vi "MatrixSwitch.vi"(8 "error in (no error)":errorcluster, 10 "Action":T1(ring), 11 "Pickering in":refnum<class "Pickering.lvclass">) -> (0 "error out":errorcluster, 2 "Continue?":bool, 3 "Pickering out":refnum<class "Pickering.lvclass">)   [LabVIEW 2019, in "Pickering.lvclass"]
uses:
  Pickering.lvclass
  InstrumentSetup.vi
  InstrControl.lvclass
panel:
  out "Display Matrix":bool[][](array[boolean])
  # "Pickering Matrix Settings"
  # "X1"
  # "X2"
  # "X3"
  # "X4"
  # "X5"
  # "X6"
  # "X7"
  # "X8"
  # "X9"
  # "X10"
  # "X11"
  # "X12"
  # "Y1"
  # "Y2"
  # "Y3"
  # "Y4"
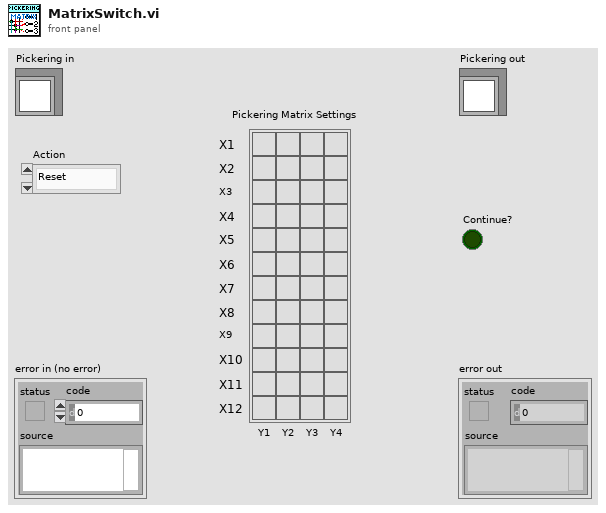
[diagram p1: front panel]
types:
  T1 = enum16{"Reset", "Ground", "Striptest Bias", "Striptest SMU", "Striptest LCR", "IV", "CV", "Interstrip Cap", "Interstrip Res", "PTP", "Implant Resistance", "Metal Resistance", "Coupling Capacitance"}
  T2 = cluster{"Matrix address":string, "Mux1 address":string, "Mux2 address":string, "Pickering":refnum<class "Pickering.lvclass">, "Matrix X Channels":cluster{"Bias Supply / SMU LO":i32, "Bias Supply / SMU HI":i32, "CV Box LO":i32, "CV Box HI":i32, "CV Box LO IN":i32, "CV Box HI IN":i32, "Volt meter LO":i32, "Volt meter HI":i32, "Mux1 C1":i32, "Mux1 C2":i32, "Mux2 C1":i32, "Mux2 C2":i32}}
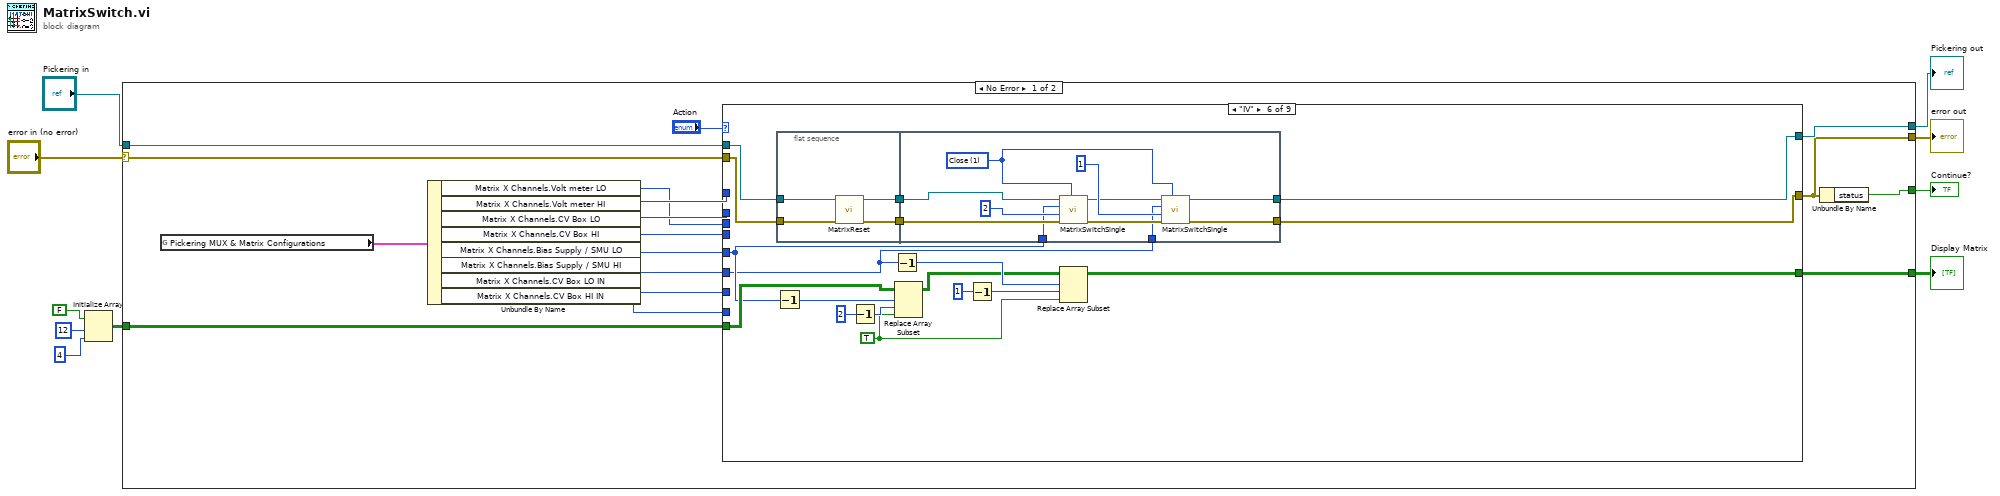
[diagram p0: block diagram]
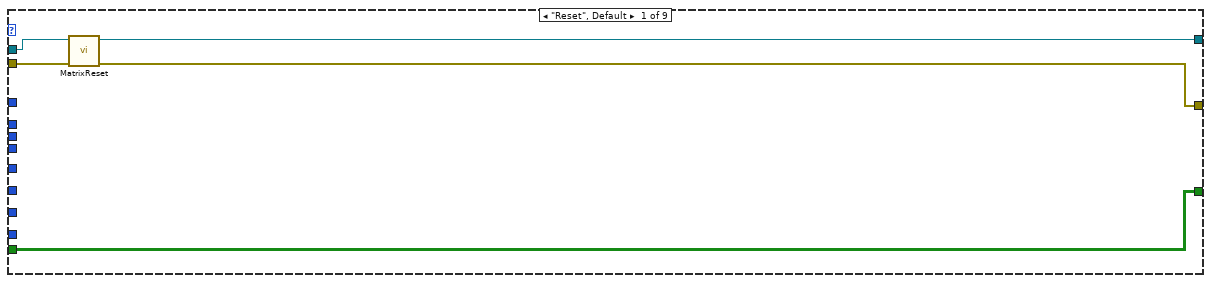
[diagram p2: hidden frame]
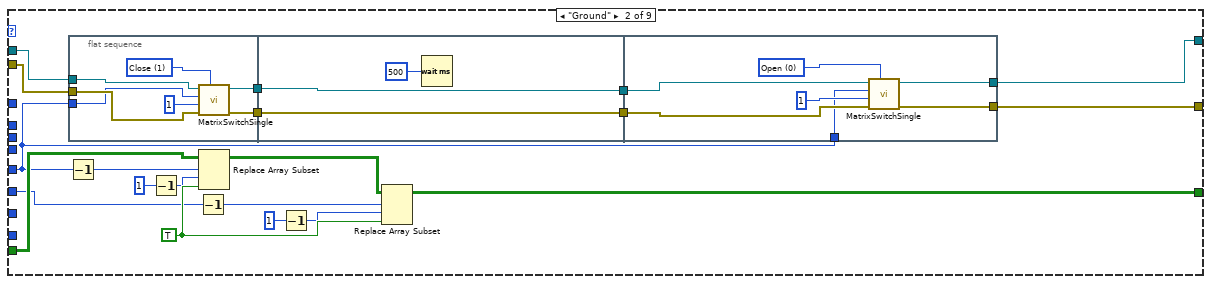
[diagram p3: hidden frame]
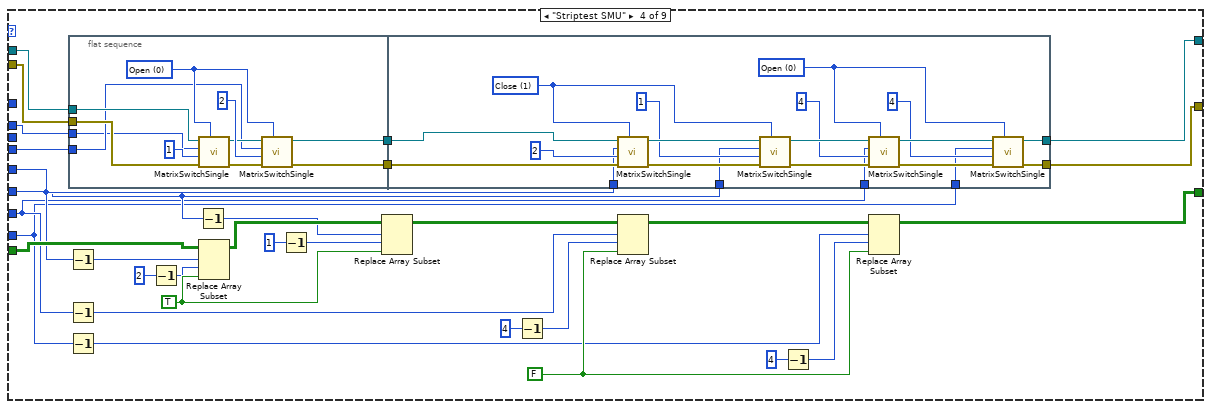
[diagram p5: hidden frame]
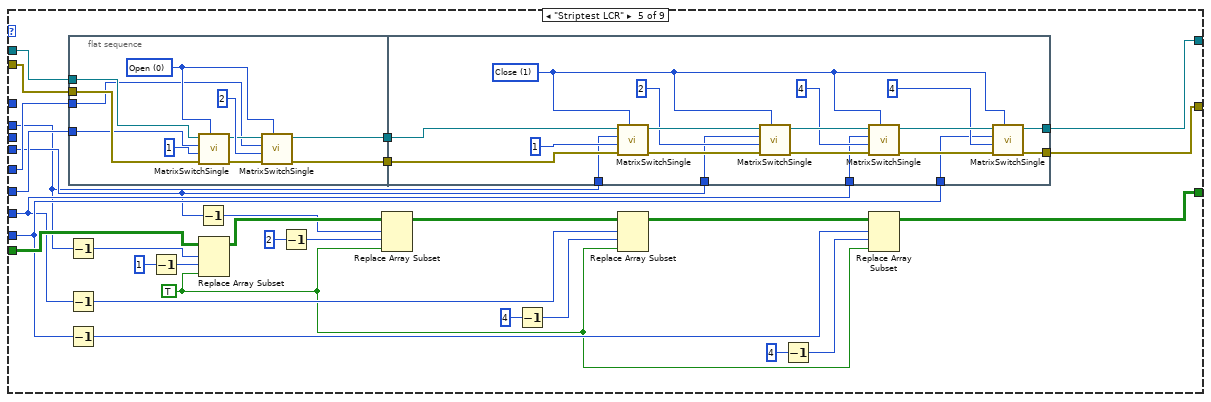
[diagram p6: hidden frame]
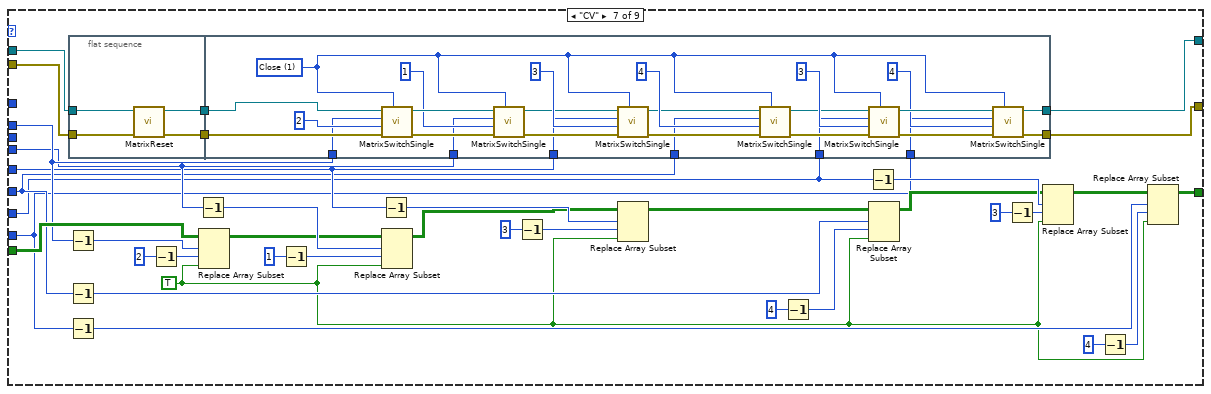
[diagram p7: hidden frame]
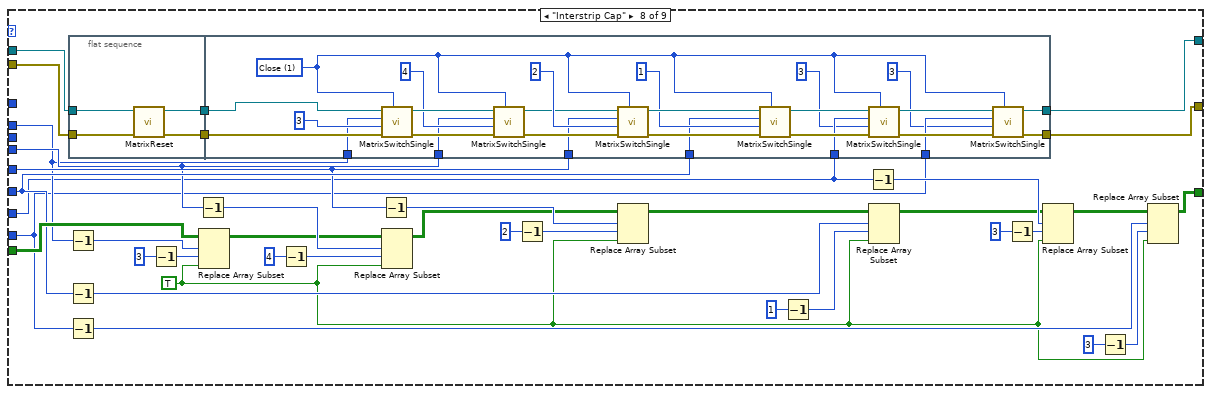
[diagram p8: hidden frame]
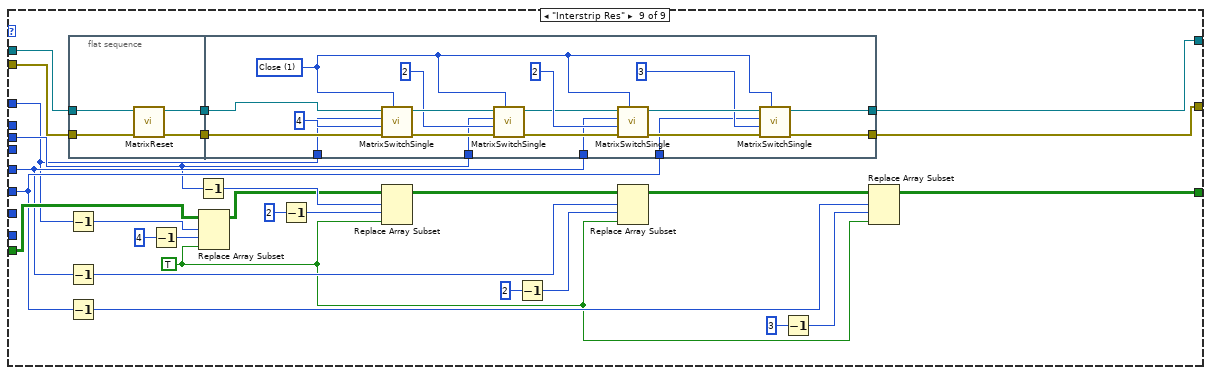
[diagram p9: hidden frame]
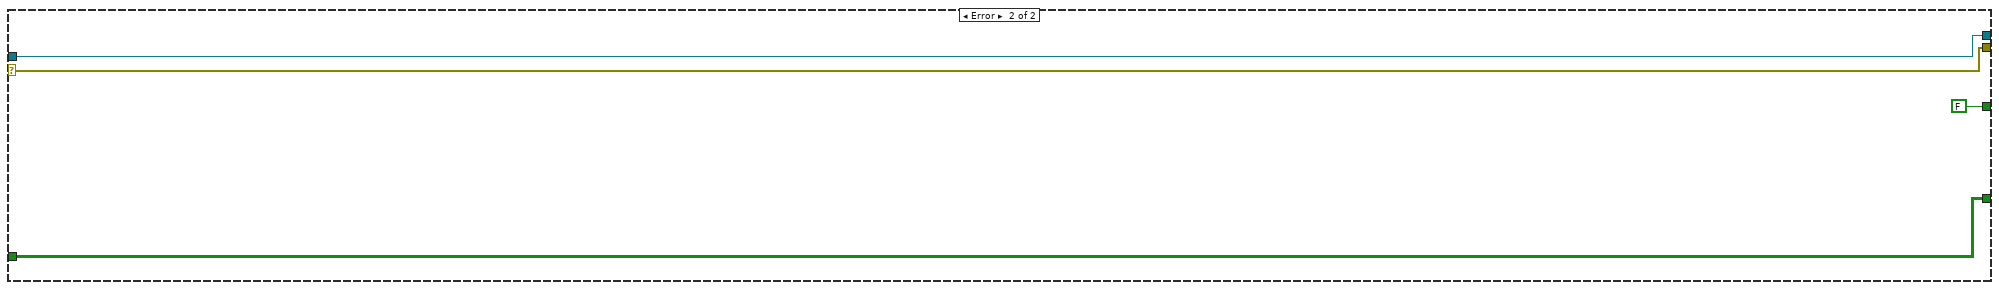
[diagram p10: hidden frame]
diagram:
  n1 = Initialize Array(FALSE, 12, 4) -> (w5:bool[][])
  n2 = case shown="No Error" "error in (no error)" {
    selector: "error in (no error)" -> [w21 w420]
    tunnel: [w24 w420] -> w2
    tunnel: [w25 w419] -> w1
    tunnel: "Pickering in" -> [w22 w419]
    tunnel: [w23 FALSE] -> w4
    tunnel: w5 -> [w27 w417]
    tunnel: [w26 w417] -> w3
    frame No Error {
      n3 = global read "InstrumentSetup.vi" "Pickering MUX & Matrix Configurations"() -> (w20:T2)
      n4 = Unbundle By Name(w20) -> ("Matrix X Channels.Volt meter LO"=w14:i32, "Matrix X Channels.Volt meter HI"=w15:i32, "Matrix X Channels.CV Box LO"=w19:i32, "Matrix X Channels.CV Box HI"=w18:i32, "Matrix X Channels.Bias Supply / SMU LO"=w12:i32, "Matrix X Channels.Bias Supply / SMU HI"=w13:i32, "Matrix X Channels.CV Box LO IN"=w17:i32, "Matrix X Channels.CV Box HI IN"=w16:i32)
      n5 = case shown="\"IV\"" "Action" {
        tunnel: w27 -> [w32 w37 w72 w90 w153 w203 w240 w320 w378]
        tunnel: [w32 w35 w72 w89 w152 w204 w241 w297 w379] -> w26
        tunnel: w21 -> [w29 w52 w71 w79 w142 w211 w239 w319 w377]
        tunnel: w22 -> [w31 w49 w70 w81 w141 w212 w238 w318 w376]
        tunnel: [w30 w46 w70 w84 w147 w200 w234 w314 w372] -> w25
        tunnel: [w28 w45 w71 w83 w146 w199 w235 w315 w373] -> w24
        tunnel: w12 -> [_ w34 _ w76 w139 w196 w231 w311 w368]
        tunnel: w13 -> [_ w33 _ w75 w140 w195 w230 w312 w369]
        tunnel: w19 -> [_ _ _ w77 w135 _ w233 w309 _]
        tunnel: w18 -> [_ _ _ w78 w136 _ w232 w310 _]
        tunnel: w17 -> [_ _ _ w74 w137 _ w229 w301 _]
        tunnel: w16 -> [_ _ _ w73 w138 _ w228 w300 _]
        tunnel: w14 -> [_ _ _ _ _ _ _ _ w367]
        tunnel: w15 -> [_ _ _ _ _ _ _ _ w366]
        frame "Reset", Default {
          n6 = call-dynamic "MatrixReset.vi"("error in (no error)"=w29, "Pickering in"=w31) -> ("error out"=w28:errorcluster, "Pickering out"=w30:refnum<class "Pickering.lvclass">)  [unwired: 8 in]
        }
        frame "Ground" {
          w43 = TRUE
          n7 = Decrement(x=w34) -> (x-1=w38:i32)
          n8 = flat-sequence {
            tunnel: w52 -> [w57]
            tunnel: [w56] -> w51
            tunnel: w49 -> [w55]
            tunnel: [w54] -> w47
            tunnel: w34 -> [w53]
            tunnel: w51 -> [w61]
            tunnel: [w61] -> w50
            tunnel: [w60] -> w48
            tunnel: w47 -> [w60]
            tunnel: w50 -> [w68]
            tunnel: w48 -> [w66]
            tunnel: [w65] -> w46
            tunnel: [w64] -> w45
            tunnel: w34 -> [w63]
            frame #0 {
              w59 = u16 1 items=["Open", "Close"] ("Switch action")
              n9 = call-dynamic "MatrixSwitchSingle.vi"("Switch action"=w59, "error in (no error)"=w57, "Matrix Y"=1, "Matrix X"=w53, "Pickering in"=w55) -> ("error out"=w56:errorcluster, "Pickering out"=w54:refnum<class "Pickering.lvclass">)  [unwired: 4 in, 1 out]
            }
            frame #1 {
              n10 = Wait (ms)(milliseconds to wait=u32 500) -> ()  [unwired: 1 out]
            }
            frame #2 {
              w69 = u16 0 items=["Open", "Close"] ("Switch action")
              n11 = call-dynamic "MatrixSwitchSingle.vi"("Switch action"=w69, "error in (no error)"=w68, "Matrix Y"=1, "Matrix X"=w63, "Pickering in"=w66) -> ("error out"=w64:errorcluster, "Pickering out"=w65:refnum<class "Pickering.lvclass">)  [unwired: 4 in, 1 out]
            }
          }
          n12 = Decrement(x=1 ("Matrix Y")) -> (x-1=w39:i32)
          n13 = Decrement(x=w33) -> (x-1=w40:i32)
          n14 = Replace Array Subset(array=w37, new element=w43, index (row)=w38, index (col)=w39) -> (w44:bool[][])
          n15 = Decrement(x=1 ("Matrix Y")) -> (x-1=w41:i32)
          n16 = Replace Array Subset(array=w44, new element=w43, index (row)=w40, index (col)=w41) -> (w35:bool[][])
        }
        frame "Striptest Bias" {
          # "Does nothing as the bias is connected directly for the Pickering GPIB switching system."
        }
        frame "Striptest SMU" {
          w103 = FALSE
          w102 = TRUE
          n17 = Decrement(x=w76) -> (x-1=w92:i32)
          n18 = Decrement(x=w74) -> (x-1=w97:i32)
          n19 = Decrement(x=w73) -> (x-1=w98:i32)
          n20 = flat-sequence {
            tunnel: [w110] -> w82
            tunnel: w81 -> [w108]
            tunnel: [w107] -> w80
            tunnel: w79 -> [w106]
            tunnel: w78 -> [w105]
            tunnel: w77 -> [w104]
            tunnel: [w123] -> w84
            tunnel: [w122] -> w83
            tunnel: w82 -> [w120]
            tunnel: w80 -> [w119]
            tunnel: w74 -> [w118]
            tunnel: w73 -> [w117]
            tunnel: w75 -> [w116]
            tunnel: w76 -> [w115]
            frame #0 {
              w109 = u16 0 items=["Open", "Close"] ("Switch action")
              n21 = call-dynamic "MatrixSwitchSingle.vi"("Switch action"=w109, "error in (no error)"=w106, "Matrix Y"=1, "Matrix X"=w104, "Pickering in"=w108) -> ("error out"=w113:errorcluster, "Pickering out"=w112:refnum<class "Pickering.lvclass">)  [unwired: 4 in, 1 out]
              n22 = call-dynamic "MatrixSwitchSingle.vi"("Switch action"=w109, "error in (no error)"=w113, "Matrix Y"=2, "Matrix X"=w105, "Pickering in"=w112) -> ("error out"=w110:errorcluster, "Pickering out"=w107:refnum<class "Pickering.lvclass">)  [unwired: 4 in, 1 out]
            }
            frame #1 {
              w121 = u16 0 items=["Open", "Close"] ("Switch action")
              w132 = u16 1 items=["Open", "Close"] ("Switch action")
              n23 = call-dynamic "MatrixSwitchSingle.vi"("Switch action"=w132, "error in (no error)"=w120, "Matrix Y"=2, "Matrix X"=w115, "Pickering in"=w119) -> ("error out"=w130:errorcluster, "Pickering out"=w133:refnum<class "Pickering.lvclass">)  [unwired: 4 in, 1 out]
              n24 = call-dynamic "MatrixSwitchSingle.vi"("Switch action"=w132, "error in (no error)"=w130, "Matrix Y"=1, "Matrix X"=w116, "Pickering in"=w133) -> ("error out"=w128:errorcluster, "Pickering out"=w129:refnum<class "Pickering.lvclass">)  [unwired: 4 in, 1 out]
              n25 = call-dynamic "MatrixSwitchSingle.vi"("Switch action"=w121, "error in (no error)"=w128, "Matrix Y"=4, "Matrix X"=w118, "Pickering in"=w129) -> ("error out"=w125:errorcluster, "Pickering out"=w126:refnum<class "Pickering.lvclass">)  [unwired: 4 in, 1 out]
              n26 = call-dynamic "MatrixSwitchSingle.vi"("Switch action"=w121, "error in (no error)"=w125, "Matrix Y"=4, "Matrix X"=w117, "Pickering in"=w126) -> ("error out"=w122:errorcluster, "Pickering out"=w123:refnum<class "Pickering.lvclass">)  [unwired: 4 in, 1 out]
            }
          }
          n27 = Decrement(x=2 ("Matrix Y")) -> (x-1=w91:i32)
          n28 = Decrement(x=w75) -> (x-1=w93:i32)
          n29 = Replace Array Subset(array=w90, new element=w102, index (row)=w92, index (col)=w91) -> (w95:bool[][])
          n30 = Decrement(x=1 ("Matrix Y")) -> (x-1=w94:i32)
          n31 = Replace Array Subset(array=w95, new element=w102, index (row)=w93, index (col)=w94) -> (w101:bool[][])
          n32 = Decrement(x=4 ("Matrix Y")) -> (x-1=w96:i32)
          n33 = Replace Array Subset(array=w101, new element=w103, index (row)=w97, index (col)=w96) -> (w100:bool[][])
          n34 = Decrement(x=4 ("Matrix Y")) -> (x-1=w99:i32)
          n35 = Replace Array Subset(array=w100, new element=w103, index (row)=w98, index (col)=w99) -> (w89:bool[][])
        }
        frame "Striptest LCR" {
          w145 = TRUE
          n36 = Decrement(x=w135) -> (x-1=w155:i32)
          n37 = Decrement(x=w137) -> (x-1=w160:i32)
          n38 = Decrement(x=w138) -> (x-1=w161:i32)
          n39 = flat-sequence {
            tunnel: [w171] -> w144
            tunnel: [w170] -> w143
            tunnel: w142 -> [w169]
            tunnel: w141 -> [w168]
            tunnel: w139 -> [w166]
            tunnel: w140 -> [w165]
            tunnel: [w184] -> w147
            tunnel: [w183] -> w146
            tunnel: w144 -> [w181]
            tunnel: w143 -> [w180]
            tunnel: w135 -> [w179]
            tunnel: w136 -> [w178]
            tunnel: w137 -> [w177]
            tunnel: w138 -> [w176]
            frame #0 {
              w167 = u16 0 items=["Open", "Close"] ("Switch action")
              n40 = call-dynamic "MatrixSwitchSingle.vi"("Switch action"=w167, "error in (no error)"=w169, "Matrix Y"=1, "Matrix X"=w165, "Pickering in"=w168) -> ("error out"=w174:errorcluster, "Pickering out"=w173:refnum<class "Pickering.lvclass">)  [unwired: 4 in, 1 out]
              n41 = call-dynamic "MatrixSwitchSingle.vi"("Switch action"=w167, "error in (no error)"=w174, "Matrix Y"=2, "Matrix X"=w166, "Pickering in"=w173) -> ("error out"=w170:errorcluster, "Pickering out"=w171:refnum<class "Pickering.lvclass">)  [unwired: 4 in, 1 out]
            }
            frame #1 {
              w182 = u16 1 items=["Open", "Close"] ("Switch action")
              n42 = call-dynamic "MatrixSwitchSingle.vi"("Switch action"=w182, "error in (no error)"=w180, "Matrix Y"=1, "Matrix X"=w179, "Pickering in"=w181) -> ("error out"=w191:errorcluster, "Pickering out"=w193:refnum<class "Pickering.lvclass">)  [unwired: 4 in, 1 out]
              n43 = call-dynamic "MatrixSwitchSingle.vi"("Switch action"=w182, "error in (no error)"=w191, "Matrix Y"=2, "Matrix X"=w178, "Pickering in"=w193) -> ("error out"=w189:errorcluster, "Pickering out"=w190:refnum<class "Pickering.lvclass">)  [unwired: 4 in, 1 out]
              n44 = call-dynamic "MatrixSwitchSingle.vi"("Switch action"=w182, "error in (no error)"=w189, "Matrix Y"=4, "Matrix X"=w177, "Pickering in"=w190) -> ("error out"=w186:errorcluster, "Pickering out"=w187:refnum<class "Pickering.lvclass">)  [unwired: 4 in, 1 out]
              n45 = call-dynamic "MatrixSwitchSingle.vi"("Switch action"=w182, "error in (no error)"=w186, "Matrix Y"=4, "Matrix X"=w176, "Pickering in"=w187) -> ("error out"=w183:errorcluster, "Pickering out"=w184:refnum<class "Pickering.lvclass">)  [unwired: 4 in, 1 out]
            }
          }
          n46 = Decrement(x=1 ("Matrix Y")) -> (x-1=w154:i32)
          n47 = Decrement(x=w136) -> (x-1=w156:i32)
          n48 = Replace Array Subset(array=w153, new element=w145, index (row)=w155, index (col)=w154) -> (w158:bool[][])
          n49 = Decrement(x=2 ("Matrix Y")) -> (x-1=w157:i32)
          n50 = Replace Array Subset(array=w158, new element=w145, index (row)=w156, index (col)=w157) -> (w164:bool[][])
          n51 = Decrement(x=4 ("Matrix Y")) -> (x-1=w159:i32)
          n52 = Replace Array Subset(array=w164, new element=w145, index (row)=w160, index (col)=w159) -> (w163:bool[][])
          n53 = Decrement(x=4 ("Matrix Y")) -> (x-1=w162:i32)
          n54 = Replace Array Subset(array=w163, new element=w145, index (row)=w161, index (col)=w162) -> (w152:bool[][])
        }
        frame "IV" {
          w206 = TRUE
          n55 = Decrement(x=w196) -> (x-1=w208:i32)
          n56 = flat-sequence {
            tunnel: w212 -> [w216]
            tunnel: w211 -> [w215]
            tunnel: [w214] -> w202
            tunnel: [w213] -> w201
            tunnel: w202 -> [w222]
            tunnel: w201 -> [w221]
            tunnel: [w220] -> w200
            tunnel: [w219] -> w199
            tunnel: w195 -> [w218]
            tunnel: w196 -> [w217]
            frame #0 {
              n57 = call-dynamic "MatrixReset.vi"("error in (no error)"=w215, "Pickering in"=w216) -> ("error out"=w213:errorcluster, "Pickering out"=w214:refnum<class "Pickering.lvclass">)  [unwired: 8 in]
            }
            frame #1 {
              w227 = u16 1 items=["Open", "Close"] ("Switch action")
              n58 = call-dynamic "MatrixSwitchSingle.vi"("Switch action"=w227, "error in (no error)"=w221, "Matrix Y"=2, "Matrix X"=w217, "Pickering in"=w222) -> ("error out"=w225:errorcluster, "Pickering out"=w224:refnum<class "Pickering.lvclass">)  [unwired: 4 in, 1 out]
              n59 = call-dynamic "MatrixSwitchSingle.vi"("Switch action"=w227, "error in (no error)"=w225, "Matrix Y"=1, "Matrix X"=w218, "Pickering in"=w224) -> ("error out"=w219:errorcluster, "Pickering out"=w220:refnum<class "Pickering.lvclass">)  [unwired: 4 in, 1 out]
            }
          }
          n60 = Decrement(x=2 ("Matrix Y")) -> (x-1=w207:i32)
          n61 = Decrement(x=w195) -> (x-1=w210:i32)
          n62 = Replace Array Subset(array=w203, new element=w206, index (row)=w208, index (col)=w207) -> (w205:bool[][])
          n63 = Decrement(x=1 ("Matrix Y")) -> (x-1=w209:i32)
          n64 = Replace Array Subset(array=w205, new element=w206, index (row)=w210, index (col)=w209) -> (w204:bool[][])
        }
        frame "CV" {
          w250 = TRUE
          n65 = Decrement(x=w233) -> (x-1=w263:i32)
          n66 = Decrement(x=w230) -> (x-1=w256:i32)
          n67 = Decrement(x=w228) -> (x-1=w255:i32)
          n68 = flat-sequence {
            tunnel: w239 -> [w269]
            tunnel: w238 -> [w268]
            tunnel: [w267] -> w237
            tunnel: [w266] -> w236
            tunnel: w237 -> [w279]
            tunnel: w236 -> [w278]
            tunnel: [w277] -> w235
            tunnel: [w276] -> w234
            tunnel: w233 -> [w275]
            tunnel: w232 -> [w274]
            tunnel: w231 -> [w273]
            tunnel: w230 -> [w272]
            tunnel: w229 -> [w271]
            tunnel: w228 -> [w270]
            frame #0 {
              n69 = call-dynamic "MatrixReset.vi"("error in (no error)"=w269, "Pickering in"=w268) -> ("error out"=w266:errorcluster, "Pickering out"=w267:refnum<class "Pickering.lvclass">)  [unwired: 8 in]
            }
            frame #1 {
              w282 = u16 1 items=["Open", "Close"] ("Switch action")
              n70 = call-dynamic "MatrixSwitchSingle.vi"("Switch action"=w282, "error in (no error)"=w278, "Matrix Y"=2, "Matrix X"=w275, "Pickering in"=w279) -> ("error out"=w284:errorcluster, "Pickering out"=w285:refnum<class "Pickering.lvclass">)  [unwired: 4 in, 1 out]
              n71 = call-dynamic "MatrixSwitchSingle.vi"("Switch action"=w282, "error in (no error)"=w284, "Matrix Y"=1, "Matrix X"=w274, "Pickering in"=w285) -> ("error out"=w280:errorcluster, "Pickering out"=w281:refnum<class "Pickering.lvclass">)  [unwired: 4 in, 1 out]
              n72 = call-dynamic "MatrixSwitchSingle.vi"("Switch action"=w282, "error in (no error)"=w280, "Matrix Y"=3, "Matrix X"=w273, "Pickering in"=w281) -> ("error out"=w295:errorcluster, "Pickering out"=w294:refnum<class "Pickering.lvclass">)  [unwired: 4 in, 1 out]
              n73 = call-dynamic "MatrixSwitchSingle.vi"("Switch action"=w282, "error in (no error)"=w295, "Matrix Y"=4, "Matrix X"=w272, "Pickering in"=w294) -> ("error out"=w287:errorcluster, "Pickering out"=w288:refnum<class "Pickering.lvclass">)  [unwired: 4 in, 1 out]
              n74 = call-dynamic "MatrixSwitchSingle.vi"("Switch action"=w282, "error in (no error)"=w287, "Matrix Y"=3, "Matrix X"=w271, "Pickering in"=w288) -> ("error out"=w290:errorcluster, "Pickering out"=w291:refnum<class "Pickering.lvclass">)  [unwired: 4 in, 1 out]
              n75 = call-dynamic "MatrixSwitchSingle.vi"("Switch action"=w282, "error in (no error)"=w290, "Matrix Y"=4, "Matrix X"=w270, "Pickering in"=w291) -> ("error out"=w277:errorcluster, "Pickering out"=w276:refnum<class "Pickering.lvclass">)  [unwired: 4 in, 1 out]
            }
          }
          n76 = Decrement(x=2 ("Matrix Y")) -> (x-1=w262:i32)
          n77 = Decrement(x=w232) -> (x-1=w265:i32)
          n78 = Replace Array Subset(array=w240, new element=w250, index (row)=w263, index (col)=w262) -> (w261:bool[][])
          n79 = Decrement(x=1 ("Matrix Y")) -> (x-1=w264:i32)
          n80 = Decrement(x=w231) -> (x-1=w258:i32)
          n81 = Replace Array Subset(array=w261, new element=w250, index (row)=w265, index (col)=w264) -> (w243:bool[][])
          n82 = Decrement(x=3 ("Matrix Y")) -> (x-1=w259:i32)
          n83 = Replace Array Subset(array=w243, new element=w250, index (row)=w258, index (col)=w259) -> (w260:bool[][])
          n84 = Decrement(x=4 ("Matrix Y")) -> (x-1=w257:i32)
          n85 = Decrement(x=w229) -> (x-1=w253:i32)
          n86 = Replace Array Subset(array=w260, new element=w250, index (row)=w256, index (col)=w257) -> (w242:bool[][])
          n87 = Decrement(x=3 ("Matrix Y")) -> (x-1=w252:i32)
          n88 = Replace Array Subset(array=w242, new element=w250, index (row)=w253, index (col)=w252) -> (w251:bool[][])
          n89 = Decrement(x=4 ("Matrix Y")) -> (x-1=w254:i32)
          n90 = Replace Array Subset(array=w251, new element=w250, index (row)=w255, index (col)=w254) -> (w241:bool[][])
        }
        frame "Interstrip Cap" {
          w302 = TRUE
          n91 = Decrement(x=w309) -> (x-1=w332:i32)
          n92 = Decrement(x=w312) -> (x-1=w329:i32)
          n93 = Decrement(x=w300) -> (x-1=w308:i32)
          n94 = flat-sequence {
            tunnel: w319 -> [w338]
            tunnel: w318 -> [w337]
            tunnel: [w336] -> w317
            tunnel: [w335] -> w316
            tunnel: w317 -> [w357]
            tunnel: w316 -> [w356]
            tunnel: [w341] -> w315
            tunnel: [w340] -> w314
            tunnel: w309 -> [w353]
            tunnel: w310 -> [w352]
            tunnel: w311 -> [w351]
            tunnel: w312 -> [w350]
            tunnel: w301 -> [w345]
            tunnel: w300 -> [w344]
            frame #0 {
              n95 = call-dynamic "MatrixReset.vi"("error in (no error)"=w338, "Pickering in"=w337) -> ("error out"=w335:errorcluster, "Pickering out"=w336:refnum<class "Pickering.lvclass">)  [unwired: 8 in]
            }
            frame #1 {
              w339 = u16 1 items=["Open", "Close"] ("Switch action")
              n96 = call-dynamic "MatrixSwitchSingle.vi"("Switch action"=w339, "error in (no error)"=w356, "Matrix Y"=3, "Matrix X"=w353, "Pickering in"=w357) -> ("error out"=w359:errorcluster, "Pickering out"=w360:refnum<class "Pickering.lvclass">)  [unwired: 4 in, 1 out]
              n97 = call-dynamic "MatrixSwitchSingle.vi"("Switch action"=w339, "error in (no error)"=w359, "Matrix Y"=4, "Matrix X"=w352, "Pickering in"=w360) -> ("error out"=w354:errorcluster, "Pickering out"=w355:refnum<class "Pickering.lvclass">)  [unwired: 4 in, 1 out]
              n98 = call-dynamic "MatrixSwitchSingle.vi"("Switch action"=w339, "error in (no error)"=w354, "Matrix Y"=2, "Matrix X"=w351, "Pickering in"=w355) -> ("error out"=w363:errorcluster, "Pickering out"=w364:refnum<class "Pickering.lvclass">)  [unwired: 4 in, 1 out]
              n99 = call-dynamic "MatrixSwitchSingle.vi"("Switch action"=w339, "error in (no error)"=w363, "Matrix Y"=1, "Matrix X"=w350, "Pickering in"=w364) -> ("error out"=w347:errorcluster, "Pickering out"=w346:refnum<class "Pickering.lvclass">)  [unwired: 4 in, 1 out]
              n100 = call-dynamic "MatrixSwitchSingle.vi"("Switch action"=w339, "error in (no error)"=w347, "Matrix Y"=3, "Matrix X"=w345, "Pickering in"=w346) -> ("error out"=w349:errorcluster, "Pickering out"=w348:refnum<class "Pickering.lvclass">)  [unwired: 4 in, 1 out]
              n101 = call-dynamic "MatrixSwitchSingle.vi"("Switch action"=w339, "error in (no error)"=w349, "Matrix Y"=3, "Matrix X"=w344, "Pickering in"=w348) -> ("error out"=w341:errorcluster, "Pickering out"=w340:refnum<class "Pickering.lvclass">)  [unwired: 4 in, 1 out]
            }
          }
          n102 = Decrement(x=3 ("Matrix Y")) -> (x-1=w331:i32)
          n103 = Decrement(x=w310) -> (x-1=w334:i32)
          n104 = Replace Array Subset(array=w320, new element=w302, index (row)=w332, index (col)=w331) -> (w330:bool[][])
          n105 = Decrement(x=4 ("Matrix Y")) -> (x-1=w333:i32)
          n106 = Decrement(x=w311) -> (x-1=w327:i32)
          n107 = Replace Array Subset(array=w330, new element=w302, index (row)=w334, index (col)=w333) -> (w313:bool[][])
          n108 = Decrement(x=2 ("Matrix Y")) -> (x-1=w326:i32)
          n109 = Replace Array Subset(array=w313, new element=w302, index (row)=w327, index (col)=w326) -> (w325:bool[][])
          n110 = Decrement(x=1 ("Matrix Y")) -> (x-1=w328:i32)
          n111 = Decrement(x=w301) -> (x-1=w306:i32)
          n112 = Replace Array Subset(array=w325, new element=w302, index (row)=w329, index (col)=w328) -> (w304:bool[][])
          n113 = Decrement(x=3 ("Matrix Y")) -> (x-1=w305:i32)
          n114 = Replace Array Subset(array=w304, new element=w302, index (row)=w306, index (col)=w305) -> (w303:bool[][])
          n115 = Decrement(x=3 ("Matrix Y")) -> (x-1=w307:i32)
          n116 = Replace Array Subset(array=w303, new element=w302, index (row)=w308, index (col)=w307) -> (w297:bool[][])
        }
        frame "Interstrip Res" {
          w370 = TRUE
          n117 = Decrement(x=w366) -> (x-1=w391:i32)
          n118 = Decrement(x=w368) -> (x-1=w386:i32)
          n119 = Decrement(x=w369) -> (x-1=w388:i32)
          n120 = flat-sequence {
            tunnel: w377 -> [w397]
            tunnel: w376 -> [w396]
            tunnel: [w395] -> w375
            tunnel: [w394] -> w374
            tunnel: w375 -> [w407]
            tunnel: w374 -> [w406]
            tunnel: [w405] -> w373
            tunnel: [w404] -> w372
            tunnel: w368 -> [w401]
            tunnel: w369 -> [w400]
            tunnel: w367 -> [w399]
            tunnel: w366 -> [w398]
            frame #0 {
              n121 = call-dynamic "MatrixReset.vi"("error in (no error)"=w397, "Pickering in"=w396) -> ("error out"=w394:errorcluster, "Pickering out"=w395:refnum<class "Pickering.lvclass">)  [unwired: 8 in]
            }
            frame #1 {
              w408 = u16 1 items=["Open", "Close"] ("Switch action")
              n122 = call-dynamic "MatrixSwitchSingle.vi"("Switch action"=w408, "error in (no error)"=w406, "Matrix Y"=4, "Matrix X"=w398, "Pickering in"=w407) -> ("error out"=w410:errorcluster, "Pickering out"=w411:refnum<class "Pickering.lvclass">)  [unwired: 4 in, 1 out]
              n123 = call-dynamic "MatrixSwitchSingle.vi"("Switch action"=w408, "error in (no error)"=w410, "Matrix Y"=2, "Matrix X"=w399, "Pickering in"=w411) -> ("error out"=w402:errorcluster, "Pickering out"=w403:refnum<class "Pickering.lvclass">)  [unwired: 4 in, 1 out]
              n124 = call-dynamic "MatrixSwitchSingle.vi"("Switch action"=w408, "error in (no error)"=w402, "Matrix Y"=2, "Matrix X"=w401, "Pickering in"=w403) -> ("error out"=w414:errorcluster, "Pickering out"=w415:refnum<class "Pickering.lvclass">)  [unwired: 4 in, 1 out]
              n125 = call-dynamic "MatrixSwitchSingle.vi"("Switch action"=w408, "error in (no error)"=w414, "Matrix Y"=3, "Matrix X"=w400, "Pickering in"=w415) -> ("error out"=w405:errorcluster, "Pickering out"=w404:refnum<class "Pickering.lvclass">)  [unwired: 4 in, 1 out]
            }
          }
          n126 = Decrement(x=4 ("Matrix Y")) -> (x-1=w390:i32)
          n127 = Decrement(x=w367) -> (x-1=w393:i32)
          n128 = Replace Array Subset(array=w378, new element=w370, index (row)=w391, index (col)=w390) -> (w389:bool[][])
          n129 = Decrement(x=2 ("Matrix Y")) -> (x-1=w392:i32)
          n130 = Replace Array Subset(array=w389, new element=w370, index (row)=w393, index (col)=w392) -> (w371:bool[][])
          n131 = Decrement(x=2 ("Matrix Y")) -> (x-1=w385:i32)
          n132 = Replace Array Subset(array=w371, new element=w370, index (row)=w386, index (col)=w385) -> (w384:bool[][])
          n133 = Decrement(x=3 ("Matrix Y")) -> (x-1=w387:i32)
          n134 = Replace Array Subset(array=w384, new element=w370, index (row)=w388, index (col)=w387) -> (w379:bool[][])
        }
      }
      n135 = Unbundle By Name(w24) -> ("status"=w23:bool)
    }
    frame Error {
    }
  }
  "error out" <- w2
  "Pickering out" <- w1
  "Display Matrix" <- w3
  "Continue?" <- w4
